vi "Ini file.vi"(7 "Command":enum16{"Init", "Read", "Write", "Close"}(ring), 8 "error in (no error)":errorcluster, 10 "Data in":string[](array[string])) -> (0 "error out":errorcluster, 2 "Data out":string[](array[string]))   [LabVIEW 2018]
uses:
  Controls/Path Command.ctl
  <vilib>/Utility/config.llb/NI_LVConfig.lvlib
  <vilib>/Utility/config.llb/Write Key (String).vi
  <vilib>/Utility/config.llb/Read Key (String).vi
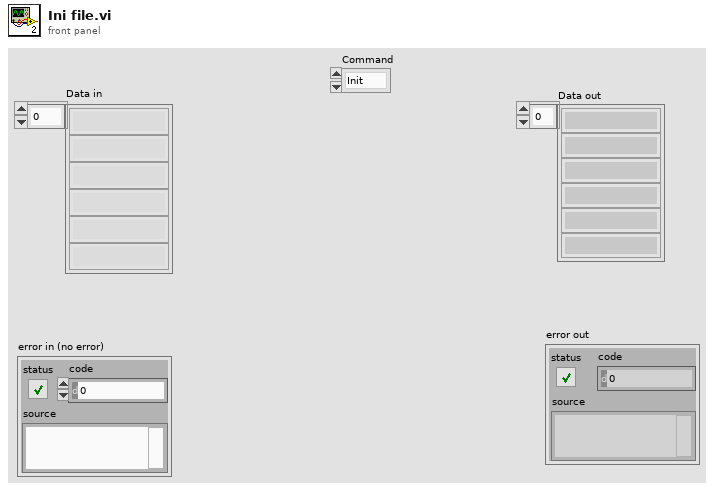
[diagram p1: front panel]
types:
  T1 = typedef "Path Command.ctl" = enum16{"Configuartion"}
  T2 = typedef "NI_LVConfig.lvlib/Config Data RefNum.ctl" = refnum<k1>
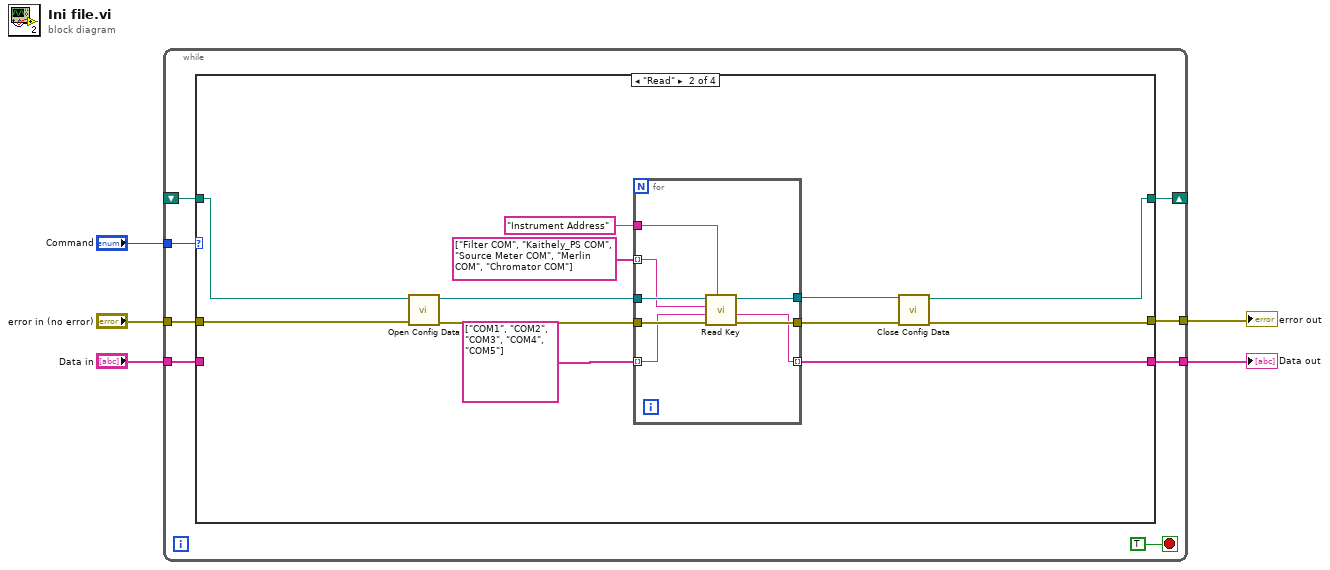
[diagram p0: block diagram]
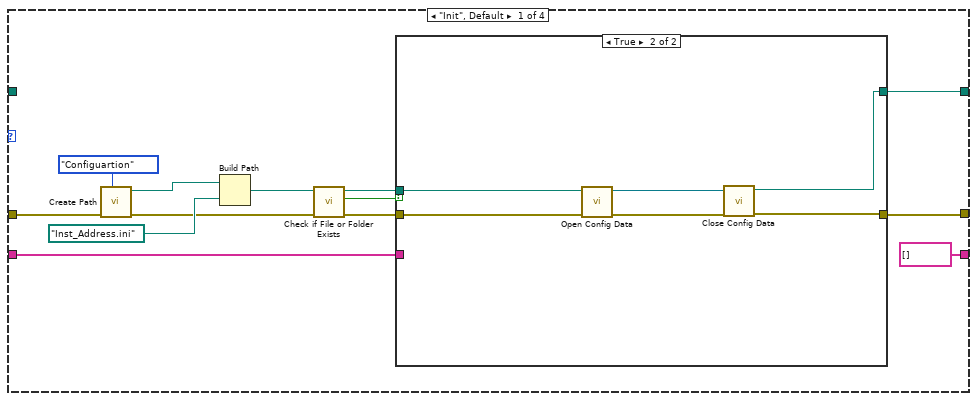
[diagram p2: hidden frame]
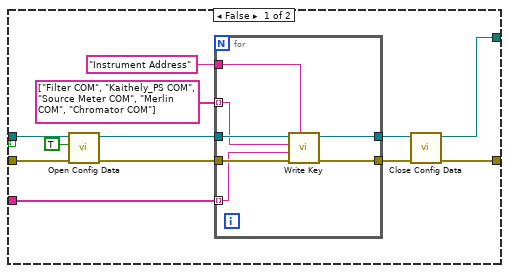
[diagram p3: hidden frame]
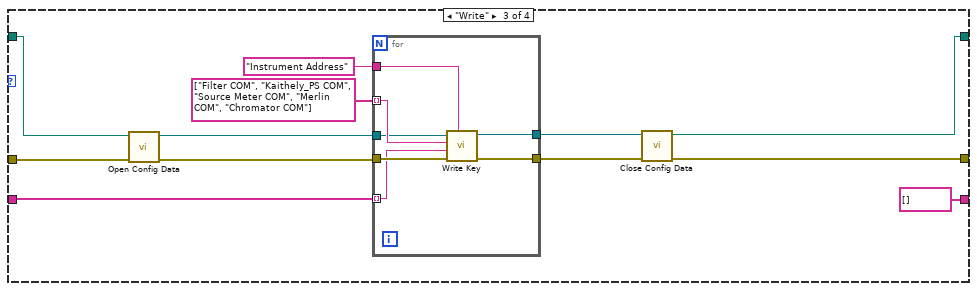
[diagram p4: hidden frame]
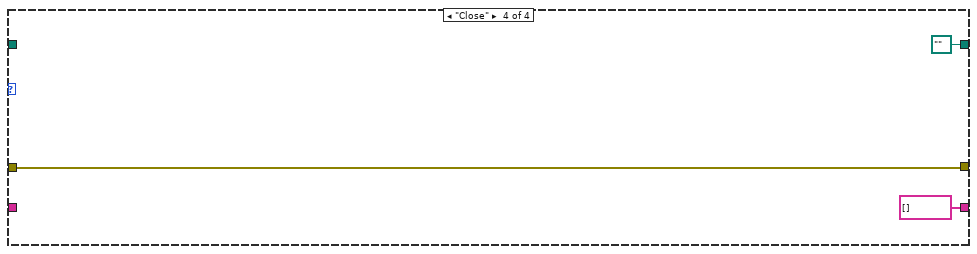
[diagram p5: hidden frame]
diagram:
  n1 = while {
    tunnel: "Command" -> [w12]
    tunnel: "error in (no error)" -> [w11]
    tunnel: [w10] -> w2
    shift-right: [w9] -> _
    shift-left: _ -> [w8]
    tunnel: "Data in" -> [w7]
    tunnel: [w6] -> w1
    stop <- TRUE stop-if-true
    n2 = case shown="\"Read\"" w12 {
      tunnel: w11 -> [w26 w63 w81 w92]
      tunnel: [w15 w55 w76 w92] -> w10
      tunnel: [w17 w54 w74 path "" ("file path")] -> w9
      tunnel: w8 -> [_ w62 w79 _]
      tunnel: w7 -> [w16 _ w82 _]
      tunnel: [string[] [] w53 string[] [] string[] []] -> w6
      frame "Init", Default {
        n3 = call "Create Path.vi"("Configuration"=Path_Command."Configuartion", "error in (no error)"=w26) -> ("error out"=w22:errorcluster, "created path"=w24:path)  [unwired: 8 in]
        n4 = Build Path(base path=w24, name or relative path=path "Inst_Address.ini") -> (appended path=w21:path)
        n5 = call <vilib>:"Check if File or Folder Exists.vi"("error in (no error)"=w22, "path"=w21) -> ("error out"=w20:errorcluster, "file or folder exists?"=w19:bool, "dup path"=w18:path)  [unwired: 7 in]
        n6 = case shown="True" w19 {
          tunnel: w20 -> [w37 w51]
          tunnel: w18 -> [w38 w50]
          tunnel: [w29 w47] -> w15
          tunnel: [w28 w46] -> w17
          tunnel: w16 -> [w32 _]
          frame False {
            n7 = call <vilib>:"Open Config Data.vi"("error in (no error)"=w37, "create file if necessary (T)"=TRUE, "configuration file path"=w38) -> ("error out"=w35:errorcluster, "refnum"=w34:T2)  [unwired: 6 in, 1 out]
            n8 = for {
              tunnel: w35 -> [w45]
              tunnel: [w43] -> w31
              tunnel: w34 -> [w44]
              tunnel: [w42] -> w30
              tunnel: string[] ["Filter COM", "Kaithely_PS COM", "Source Meter COM", "Merlin COM", "Chromator COM"] -> [w41] mode=indexing
              tunnel: w32 -> [w40] mode=indexing
              tunnel: "Instrument Address" ("section") -> [w39]
              n9 = call-poly <vilib>:"Write Key.vi"("section"=w39, "error in (no error)"=w45, "value"=w40, "key"=w41, "refnum"=w44) -> ("error out"=w43:errorcluster, "refnum out"=w42:T2)  [unwired: 4 in, 1 out]
            }
            n10 = call <vilib>:"Close Config Data.vi"("error in (no error)"=w31, "refnum"=w30) -> ("error out"=w29:errorcluster, "file path"=w28:path)  [unwired: 8 in]
          }
          frame True {
            n11 = call <vilib>:"Open Config Data.vi"("error in (no error)"=w51, "configuration file path"=w50) -> ("error out"=w49:errorcluster, "refnum"=w48:T2)  [unwired: 7 in, 1 out]
            n12 = call <vilib>:"Close Config Data.vi"("error in (no error)"=w49, "refnum"=w48) -> ("error out"=w47:errorcluster, "file path"=w46:path)  [unwired: 8 in]
          }
        }
      }
      frame "Read" {
        n13 = call <vilib>:"Open Config Data.vi"("error in (no error)"=w63, "configuration file path"=w62) -> ("error out"=w59:errorcluster, "refnum"=w58:T2)  [unwired: 7 in, 1 out]
        n14 = for {
          tunnel: string[] ["Filter COM", "Kaithely_PS COM", "Source Meter COM", "Merlin COM", "Chromator COM"] -> [w69] mode=indexing
          tunnel: "Instrument Address" ("section") -> [w68]
          tunnel: w59 -> [w71]
          tunnel: w58 -> [w70]
          tunnel: string[] ["COM1", "COM2", "COM3", "COM4", "COM5"] ("Data in") -> [w67] mode=indexing
          tunnel: [w66] -> w57
          tunnel: [w65] -> w56
          tunnel: [w64] -> w53 mode=indexing
          n15 = call-poly <vilib>:"Read Key.vi"("section"=w68, "error in (no error)"=w71, "default value"=w67, "key"=w69, "refnum"=w70) -> ("error out"=w66:errorcluster, "value"=w64:string, "refnum out"=w65:T2)  [unwired: 3 in, 1 out]
        }
        n16 = call <vilib>:"Close Config Data.vi"("error in (no error)"=w57, "refnum"=w56) -> ("error out"=w55:errorcluster, "file path"=w54:path)  [unwired: 8 in]
      }
      frame "Write" {
        n17 = call <vilib>:"Open Config Data.vi"("error in (no error)"=w81, "configuration file path"=w79) -> ("error out"=w80:errorcluster, "refnum"=w78:T2)  [unwired: 7 in, 1 out]
        n18 = for {
          tunnel: w80 -> [w90]
          tunnel: [w89] -> w77
          tunnel: [w88] -> w75
          tunnel: string[] ["Filter COM", "Kaithely_PS COM", "Source Meter COM", "Merlin COM", "Chromator COM"] -> [w87] mode=indexing
          tunnel: w82 -> [w86] mode=indexing
          tunnel: w78 -> [w85]
          tunnel: "Instrument Address" ("section") -> [w84]
          n19 = call-poly <vilib>:"Write Key.vi"("section"=w84, "error in (no error)"=w90, "value"=w86, "key"=w87, "refnum"=w85) -> ("error out"=w89:errorcluster, "refnum out"=w88:T2)  [unwired: 4 in, 1 out]
        }
        n20 = call <vilib>:"Close Config Data.vi"("error in (no error)"=w77, "refnum"=w75) -> ("error out"=w76:errorcluster, "file path"=w74:path)  [unwired: 8 in]
      }
      frame "Close" {
      }
    }
  }
  "error out" <- w2
  "Data out" <- w1
